vi "Word Easy Table.vi"   [LabVIEW 2010, in "NI_ReportGenerationToolkit.lvlib"]
doc: "Inserts and formats a table into a Microsoft Word report. The data type you wire to the <B>data</B> input determines the polymorphic instance to use."
uses:
  <vilib>/addons/_office/NI_ReportGenerationToolkit.lvlib
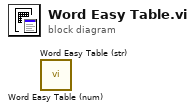
[diagram p0: block diagram]
diagram:
  n1 = call "Word Easy Table (num).vi"() -> ()  [unwired: 13 in, 3 out]
  n2 = call "Word Easy Table (str).vi"() -> ()  [unwired: 13 in, 3 out]
